vi "Teleop_Calc_Climb.vi"(11 "Teleop Local Data in":T1) -> (3 "Teleop Local Data out":T1)   [LabVIEW 2016]
uses:
  Typedefs/typedef_cluster_Teleop Local Data.ctl
  Typedefs/typedef_enum_Joystick Buttons.ctl
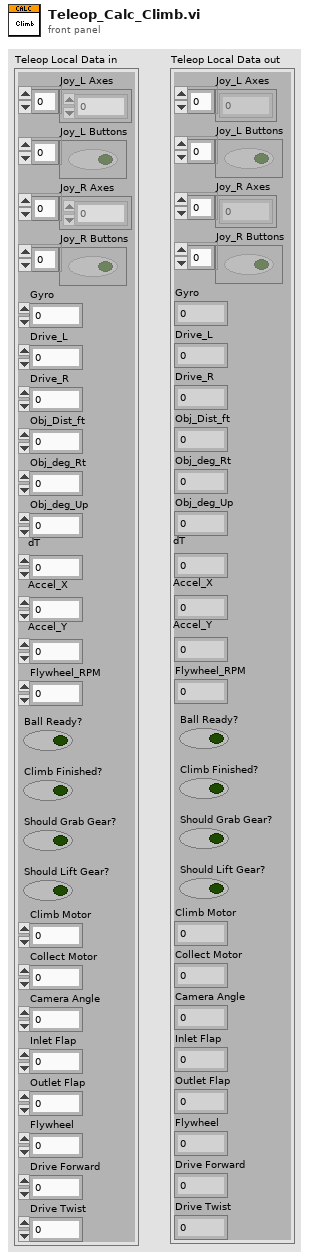
[diagram p1: front panel]
types:
  T1 = typedef "typedef_cluster_Teleop Local Data.ctl" = cluster{"Joy_L Axes":dbl[], "Joy_L Buttons":bool[], "Joy_R Axes":dbl[], "Joy_R Buttons":bool[], "Gyro":dbl, "Drive_L":i32, "Drive_R":i32, "Obj_Dist_ft":dbl, "Obj_deg_Rt":dbl, "Obj_deg_Up":dbl, "dT":dbl, "Accel_X":dbl, "Accel_Y":dbl, "Flywheel_RPM":dbl, "Ball Ready?":bool, "Climb Finished?":bool, "Should Grab Gear?":bool, "Should Lift Gear?":bool, "Climb Motor":dbl, "Collect Motor":dbl, "Camera Angle":dbl, "Inlet Flap":dbl, "Outlet Flap":dbl, "Flywheel":dbl, "Drive Forward":dbl, "Drive Twist":dbl}
  T2 = typedef "typedef_enum_Joystick Buttons.ctl" = enum16{"Trigger", "Thumb", "Top3", "Top4", "Top5", "Top6", "Low7", "Low8", "Low9", "Low10", "Low11", "Low12", "Hat0", "Hat1", "Hat2", "Hat3", "Hat4", "Hat5", "Hat6", "Hat7", "Hat8"}
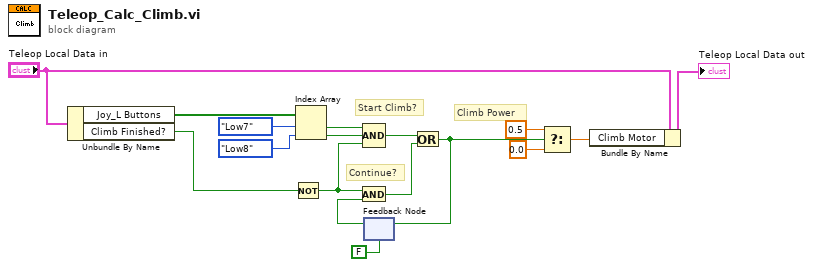
[diagram p0: block diagram]
diagram:
  # "Climb Power"
  # "Continue?"
  # "Start Climb?"
  n1 = Unbundle By Name("Teleop Local Data in") -> ("Joy_L Buttons"=w17:bool[], "Climb Finished?"=w13:bool)
  n2 = Not(x=w13) -> (.not. x?=w9:bool)
  n3 = Index Array(array=w17, index #1=typedef_enum_Joystick_Buttons."Low7" ("Joystick Buttons"), index #2=typedef_enum_Joystick_Buttons."Low8" ("Joystick Buttons")) -> (element #1=w15:bool, element #2=w14:bool)
  n4 = Compound Arithmetic op=AND(w15, w14, w9) -> (w12:bool)
  n5 = feedback #1(FALSE) -> (w10:bool)
  n6 = And(x=w9, y=w10) -> (x .and. y?=w11:bool)
  n7 = Or(x=w12, y=w11) -> (x .or. y?=w5:bool)
  n8 = feedback-in #1(w5) -> ()
  n9 = Select(t=0.5, s=w5, f=0.0) -> (s? t:f=w6:dbl)
  n10 = Bundle By Name(cluster="Teleop Local Data in", "Climb Motor"=w6) -> (→"Teleop Local Data out":T1)
